vi "test.vi"() -> ()   [LabVIEW 2020]
panel:
  out "data out":i32
  out "output array":cluster{i32, i64}[](array[cluster])
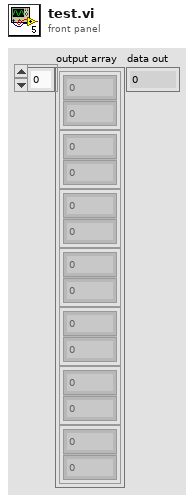
[diagram p1: front panel]
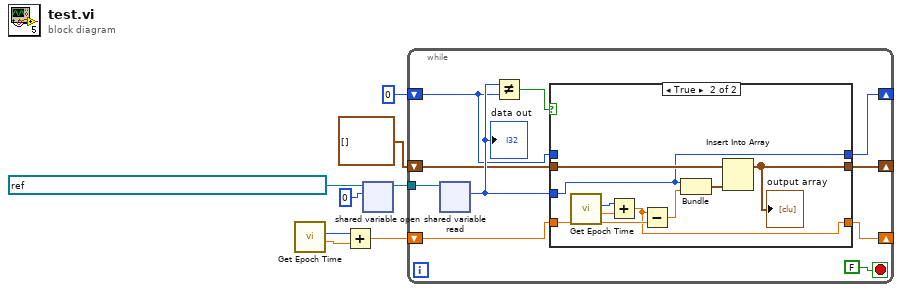
[diagram p0: block diagram]
diagram:
  n1 = call <vilib>:"Get Epoch Time.vi"() -> ("Fractional Second"=w2:dbl, "Epoch Time (s)"=w3:i64)  [unwired: 9 in, 1 out]
  n2 = Add(x=w3, y=w2) -> (x+y=w1:dbl)
  n3 = shared-variable-open(refnum<k21> "ni.var.psp://my computer/elyse_variables/elyse_counts" ("shared variable refnum in"), 0) -> (w6:refnum<k21>)  [unwired: 2 in, 1 out]
  n4 = while {
    tunnel: w6 -> [w18]
    shift-right: [w12] -> _
    shift-left: 0 -> [w15]
    shift-right: [w13] -> _
    shift-left: cluster{i32, i64}[] [] -> [w14]
    shift-right: [w9] -> _
    shift-left: w1 -> [w10]
    stop <- FALSE stop-if-true
    n5 = shared-variable-read(w18) -> (w16:i32)  [unwired: 1 in, 3 out]
    "data out" <- w16
    n6 = Not Equal?(x=w16, y=w15) -> (x != y?=w17:bool)
    n7 = case shown="True" w17 {
      tunnel: w16 -> [_ w26]
      tunnel: w15 -> [w20 _]
      tunnel: w10 -> [w19 w25]
      tunnel: w14 -> [w21 w28]
      tunnel: [w21 w27] -> w13
      tunnel: [w20 w26] -> w12
      tunnel: [w19 w22] -> w9
      frame False {
      }
      frame True {
        n8 = call <vilib>:"Get Epoch Time.vi"() -> ("Fractional Second"=w23:dbl, "Epoch Time (s)"=w24:i64)  [unwired: 9 in, 1 out]
        n9 = Add(x=w24, y=w23) -> (x+y=w22:dbl)
        n10 = Subtract(x=w22, y=w25) -> (x-y=w30:dbl)
        n11 = Bundle(w26, w30) -> (w29:cluster{i32, dbl})  [unwired: 1 in]
        n12 = Insert Into Array(array=w28, new element=w29) -> (w27:cluster{i32, i64}[])  [unwired: 1 in]
        "output array" <- w27
      }
    }
  }
